vi "generuj wykres XY.vi"(6 "Przebiegi Wfm":waveform(dbl)[](array[waveform]), 8 "error in (no error)":errorcluster, 11 "Wykresy out":string[](array[string])) -> (0 "error out":errorcluster, 2 "output cluster":cluster{"Y":dbl[], "Y":dbl[]})   [LabVIEW 2014]
doc: "Generuje wykres XY na podstawie\nwybranych przebiegów"
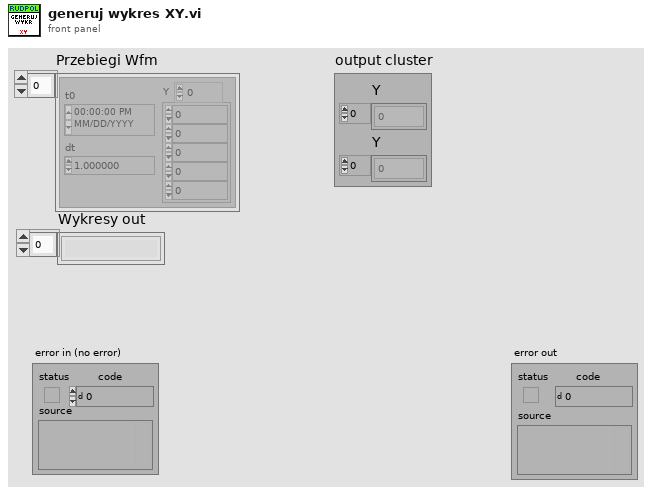
[diagram p1: front panel]
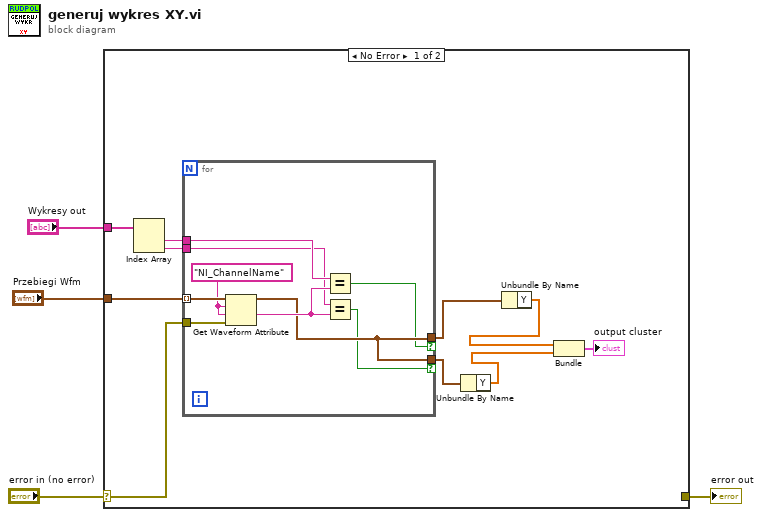
[diagram p0: block diagram]
diagram:
  n1 = case shown="No Error" "error in (no error)" {
    selector: "error in (no error)" -> [w10 w24]
    tunnel: [_ w24] -> w3
    tunnel: "Przebiegi Wfm" -> [w14 _]
    tunnel: "Wykresy out" -> [w13 _]
    frame No Error {
      n2 = Index Array(array=w13) -> (element #1=w12:string, element #2=w11:string)  [unwired: 2 in]
      n3 = for {
        tunnel: w14 -> [w23] mode=indexing
        tunnel: w12 -> [w19]
        tunnel: w11 -> [w18]
        tunnel: w10 -> [w22]
        tunnel: [w17] -> w9 if=w16
        tunnel: [w17] -> w7 if=w15
        w21 = "NI_ChannelName" ("name")
        n4 = Get Waveform Attribute(4:w22, 5:w21, 6:w21, 7:w23) -> (1:w20:string, 3:w17:waveform(dbl))  [unwired: 2 out]
        n5 = Equal?(x=w19, y=w20) -> (x = y?=w16:bool)
        n6 = Equal?(x=w18, y=w20) -> (x = y?=w15:bool)
      }
      n7 = Unbundle By Name(w7) -> ("Y"=w6:dbl[])
      n8 = Unbundle By Name(w9) -> ("Y"=w8:dbl[])
      n9 = Bundle("Y"=w8, "Y"=w6) -> (→"output cluster":cluster{"Y":dbl[], "Y":dbl[]})  [unwired: 1 in]
    }
    frame Error {
    }
  }
  "error out" <- w3
